vi "ECG Data File.vi"(8 "error in":errorcluster, 9 "Vref":dbl, 10 "CONFIG1":T1 caption="Configuration Register 1 (CONFIG1)", 11 "Working Path":path) -> (0 "error out":errorcluster, 3 "Temp File Path":path)   [LabVIEW 2010]
uses:
  Controls/Register/TYP_Reg_CONFIG1.ctl
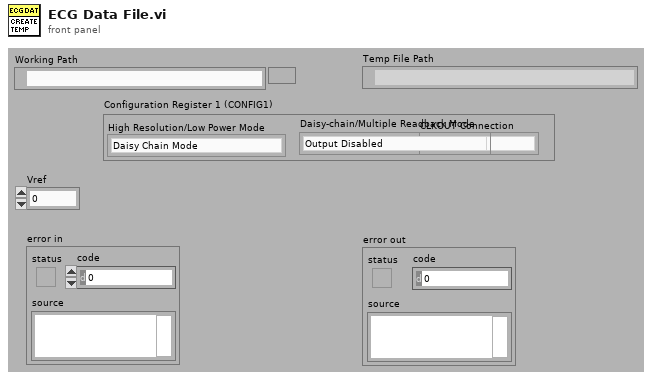
[diagram p1: front panel]
types:
  T1 = typedef "TYP_Reg_CONFIG1.ctl" = cluster{"DAISY_EN":enum16{"Daisy Chain Mode", "Multiple Readback Mode"}, "CLK_EN":enum16{"Output Disabled", "Output Enabled"}, "DR":enum16{"f(MOD) /16", "f(MOD) /32", "f(MOD) /64", "f(MOD) /128", "f(MOD) /256", "f(MOD) /512", "f(MOD) /1024"}}
  T2 = enum16{"open", "replace", "create", "open or create", "replace or create", "replace or create with confirmation"}
  T3 = enum16{"f(MOD) /16", "f(MOD) /32", "f(MOD) /64", "f(MOD) /128", "f(MOD) /256", "f(MOD) /512", "f(MOD) /1024"}
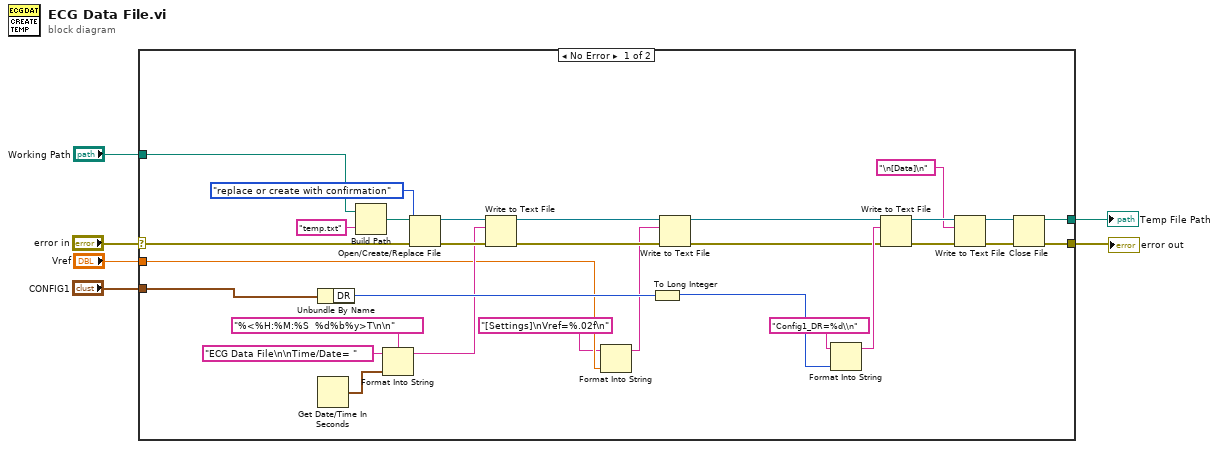
[diagram p0: block diagram]
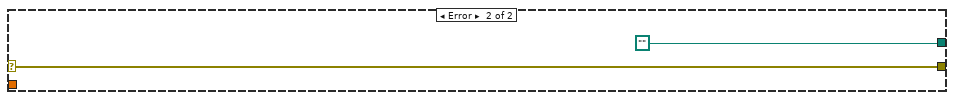
[diagram p2: hidden frame]
diagram:
  n1 = case shown="No Error" "error in" {
    selector: "error in" -> [w31 w38]
    tunnel: [w12 path ""] -> w6
    tunnel: "Working Path" -> [w36 _]
    tunnel: [w11 w38] -> w4
    tunnel: "Vref" -> [w20 _]
    tunnel: "CONFIG1" -> [w34 _]
    frame No Error {
      n2 = Unbundle By Name(w34) -> ("DR"=w33:T3)
      n3 = Get Date/Time In Seconds() -> (seconds since 1Jan1904=w27:timestamp)
      n4 = Build Path(base path=w36, name or relative path="temp.txt") -> (appended path=w32:path)
      n5 = Format Into String(format string="%<%H:%M:%S  %d%b%y>T\n\n" ("time format string (%c)"), initial string="ECG Data File\n\nTime/Date= ", w27) -> (resulting string=w24:string)  [unwired: 1 in, 1 out]
      n6 = Open/Create/Replace File(file path (use dialog)=w32, error in=w31, operation (0:open)=T2."replace or create with confirmation") -> (refnum out=w28:refnum<file>, error out=w29:errorcluster)  [unwired: 4 out]
      n7 = Write to Text File(file (use dialog)=w28, text=w24, error in=w29) -> (refnum out=w23:refnum<file>, error out=w22:errorcluster)  [unwired: 2 out]
      n8 = Format Into String(format string="[Settings]\nVref=%.02f\n" ("time format string (%c)"), w20) -> (resulting string=w21:string)  [unwired: 2 in, 1 out]
      n9 = To Long Integer(number=w33) -> (32bit integer=w17:i32)
      n10 = Write to Text File(file (use dialog)=w23, text=w21, error in=w22) -> (refnum out=w8:refnum<file>, error out=w7:errorcluster)  [unwired: 2 out]
      n11 = Format Into String(format string="Config1_DR=%d\\n" ("section"), w17) -> (resulting string=w16:string)  [unwired: 2 in, 1 out]
      n12 = Write to Text File(file (use dialog)=w8, text=w16, error in=w7) -> (refnum out=w14:refnum<file>, error out=w15:errorcluster)  [unwired: 2 out]
      n13 = Write to Text File(file (use dialog)=w14, text="\n[Data]\n", error in=w15) -> (refnum out=w13:refnum<file>, error out=w10:errorcluster)  [unwired: 2 out]
      n14 = Close File(refnum=w13, error in=w10) -> (path=w12:path, error out=w11:errorcluster)
    }
    frame Error {
    }
  }
  "Temp File Path" <- w6
  "error out" <- w4
